vi "Process.vi"(8 "error in":errorcluster, 11 "Plugin in":refnum<class "Analog Tachometer Process.lvclass">) -> (0 "error out":errorcluster, 3 "Plugin out":refnum<class "Analog Tachometer Process.lvclass">)   [LabVIEW 2025, in "Analog Tachometer Process.lvlib" / "Analog Tachometer Process.lvclass"]
uses:
  Analog Tachometer Process.lvclass
  C:/Program Files/National Instruments/LabVIEW 2025/vi.lib/FlexLogger/SDK/PluginSDK.lvlibp/PEFClasses/SDK/Plugin/Plugin.lvclass
  Analog Tachometer Process.lvclass/Analog Tachometer Process.ctl
  <vilib>/addons/Sound and Vibration/Order Analysis/Tach Process/SVPO Analog Tacho Process (1 Ch DBL WDT) with IC.vi
  <vilib>/addons/Sound and Vibration/Order Analysis/Tach Process/SVPO Analog Tacho Process (1 Ch DBL Array) with IC.vi
  <vilib>/addons/Sound and Vibration/Order Analysis/Tach Process/SubVIs/oa_Convert Pulse Positions to Speed (No State).vi
  <vilib>/addons/Sound and Vibration/Order Analysis/Tach Process/SubVIs/sv_Edge Detection (1 Tach) with IC.vi
  <vilib>/addons/Sound and Vibration/Order Analysis/Tach Process/SubVIs/oa_Analog Tacho Hysteresis(1 Channel) with IC.vi
  <vilib>/addons/_NISVFA/_Shared subVIs/Common/SV Buffer Array (No State) (DBL).vi
  <vilib>/addons/Sound and Vibration/Order Analysis/Tach Process/SubVIs/OAT Cross Point Detection.vi
  <vilib>/addons/_NISVFA/_Shared subVIs/Common/svc_Get Array Subset (Index).vi
  <vilib>/Analysis/8numeric.llb/Threshold Detector.vi
  <vilib>/addons/_NISVFA/_Shared subVIs/Common/svc_Coerce Index and Length.vi
  <vilib>/addons/_NISVFA/_Shared subVIs/Common/svc_Conditional Merge Error.vi
  <vilib>/FlexLogger/SDK/PluginSDK.lvlibp/PEFClasses/SDK/Plugin/DataHelpers/Write 1D DBL (NChan 1Sample).vi
  C:/Program Files/National Instruments/LabVIEW 2025/vi.lib/FlexLogger/SDK/PluginSDK.lvlibp/PEFClasses/SDK/Processing Element/Processing Element.lvclass
  C:/dev/dsb/niflexlogger-plugins/PDK plugins/Analog Tachometer Process/source/Analog Tachometer Process/Analog Tachometer Process.lvclass
  <vilib>/FlexLogger/SDK/PluginSDK.lvlibp/PEFClasses/SDK/Plugin/Plugin.lvclass
  <vilib>/addons/Sound and Vibration/Order Analysis/Tach Process/SoundVib_TachProcess.lvlib
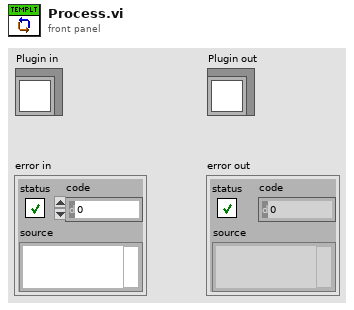
[diagram p1: front panel]
types:
  T1 = typedef "svc_Analog Tacho State.ctl" = cluster{"hysteresis state":dbl, "edge detection state":cluster{"x[n]":dbl[], "size":dbl}, "pulse to speed state":cluster{"pulse positions":dbl[], "elapsed time":dbl}}
  T2 = typedef "OAT Position Info.ctl" = cluster{"positions [s]":dbl[], "samples/rev":dbl}
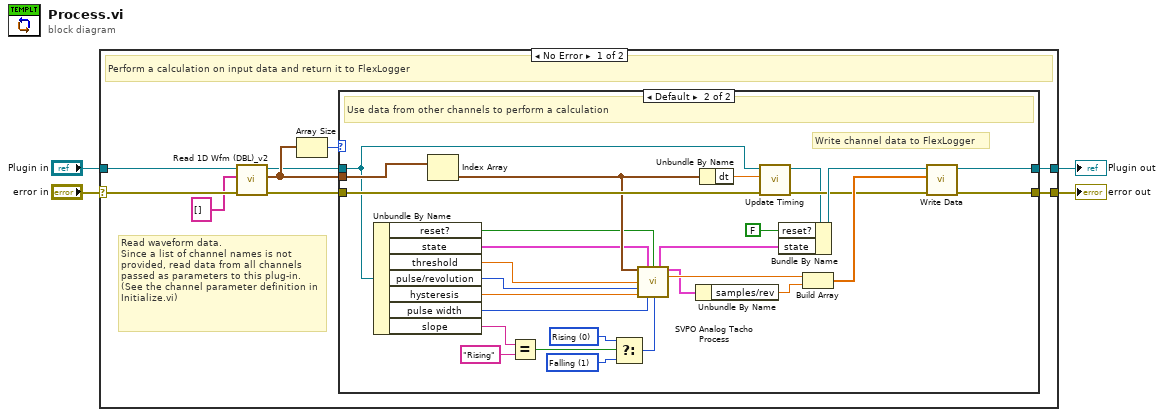
[diagram p0: block diagram]
diagram:
  n1 = case shown="No Error" "error in" {
    selector: "error in" -> [w12 w44]
    tunnel: [w10 w45] -> w1
    tunnel: "Plugin in" -> [w13 w45]
    tunnel: [w11 w44] -> w2
    frame No Error {
      # "Read waveform data.\nSince a list of channel names is not provided, read data from all channels passed as parameters to this plug-in.\n(See the channel parameter definition in Initialize.vi)"
      # "Perform a calculation on input data and return it to FlexLogger"
      n2 = call <vilib>:"Read 1D Wfm (DBL)_v2.vi"("error in (no error)"=w12, "Unique Identifiers (empty = all)"=string[] [] ("Unique Channel Identifers (empty = all)"), "Plugin in"=w13) -> ("error out"=w7:errorcluster, "Data"=w9:waveform(dbl)[], "Plugin out"=w5:refnum<class "Analog Tachometer Process.lvclass">)  [unwired: 5 in, 1 out]
      n3 = Array Size(array=w9) -> (size(s)=w8:i32)
      n4 = case shown="Default" w8 {
        tunnel: w9 -> [_ w43]
        tunnel: [w14 w42] -> w11
        tunnel: [w15 w41] -> w10
        tunnel: w5 -> [w15 w20]
        tunnel: w7 -> [w14 w24]
        frame 0 {
          # "No channels sending data to the plugin"
        }
        frame Default {
          w32 = u16 0 items=["Rising", "Falling"] ("slope (Rising)")
          w33 = u16 1 items=["Rising", "Falling"] ("slope (Rising)")
          # "Write channel data to FlexLogger"
          # "Use data from other channels to perform a calculation"
          n5 = Unbundle By Name(w20) -> ("reset?"=w19:bool, "state"=w18:T1, "threshold"=w39:dbl, "pulse/revolution"=w21:i32, "hysteresis"=w38:dbl, "pulse width"=w40:i32, "slope"=w22:string)
          n6 = Index Array(array=w43) -> (element=w23:waveform(dbl))  [unwired: 1 in]
          n7 = Equal?(x=w22, y="Rising" ("x")) -> (x = y?=w34:bool)
          n8 = Select(t=w32, s=w34, f=w33) -> (s? t:f=w31:u16)
          n9 = call-poly <vilib>:"SVPO Analog Tacho Process.vi"("analog tacho signal"=w23, "initial conditions"=w18, "reset? (F)"=w19, "threshold"=w39, "pulse/revolution (1)"=w21, "hysteresis (0)"=w38, "pulse width (2)"=w40, "slope (Rising)"=w31) -> ("final conditions"=w16:T1, "speed position info"=w29:T2, "current speed [RPM]"=w35:dbl)  [unwired: 5 in]
          n10 = Unbundle By Name(w29) -> ("samples/rev"=w28:dbl)
          n11 = Unbundle By Name(w23) -> ("dt"=w26:dbl)
          n12 = call "Update Timing.vi"("error in (no error)"=w24, "dt(sec)"=w26, "Analog Tachometer in"=w20) -> ("error out"=w27:errorcluster, "Analog Tachometer out"=w25:refnum<class "Analog Tachometer Process.lvclass">)  [unwired: 7 in]
          n13 = Bundle By Name(cluster=w25, "reset?"=FALSE, "state"=w16) -> (w36:refnum<class "Analog Tachometer Process.lvclass">)
          n14 = Build Array(w35, w28) -> (w37:dbl[])
          n15 = call-poly <vilib>:"Write Data.vi"("error in (no error)"=w27, "Data"=w37, "Plugin in"=w36) -> ("error out"=w42:errorcluster, "Plugin out"=w41:refnum<class "Analog Tachometer Process.lvclass">)  [unwired: 7 in]
        }
      }
    }
    frame Error {
    }
  }
  "error out" <- w2
  "Plugin out" <- w1
